vi "Read HackRF.vi"(8 "error in (no error)":errorcluster, 10 "Samples":i32, 11 "HRF_Device":refnum<class "HRF_Device.lvclass">) -> (0 "error out":errorcluster, 2 "Array":u8[](array[numeric]), 3 "HRF_Device out":refnum<class "HRF_Device.lvclass">)   [LabVIEW 2020, in "HRF_Device.lvclass"]
uses:
  HRF_Device.lvclass
  HRF_Device.lvclass/HRF_Device.ctl
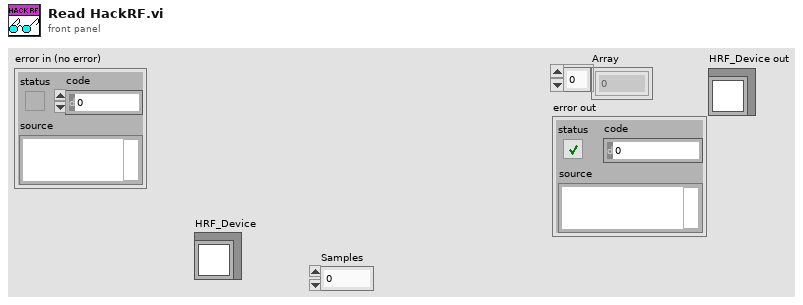
[diagram p1: front panel]
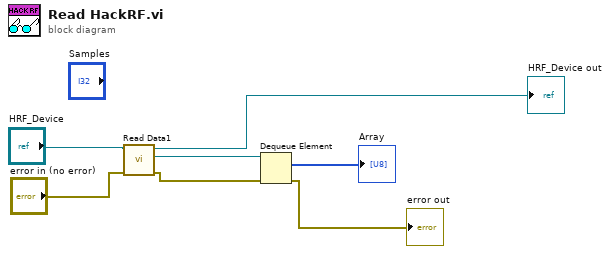
[diagram p0: block diagram]
diagram:
  n1 = call "Read Data1.vi"("error in (no error)"="error in (no error)", "HRF_Device in"="HRF_Device") -> ("error out"=w2:errorcluster, "Data"=w4:refnum<queue>, "HRF_Device out"=→"HRF_Device out":refnum<class "HRF_Device.lvclass">)  [unwired: 7 in]
  n2 = Dequeue Element(queue=w4, error in (no error)=w2) -> (element=→"Array":i32[], error out=→"error out":errorcluster)  [unwired: 1 in, 2 out]
